vi "JLINKARM Select IP.vi"(10 "Port":i32, 11 "sHost":string) -> (3 "function return":i8)   [LabVIEW 2011, in "JLinkARM.lvlib"]
doc: "JLINKARMDLL_API char JLINKARM_SelectIP (const char* sHost, int Port);"
uses:
  Lib/JLinkARM.lvlib
  JLinkARM.dll
panel:
  out "error out":errorcluster
  in  "error in (no error)":errorcluster
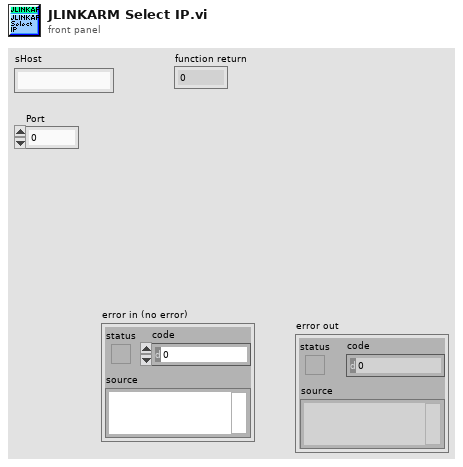
[diagram p1: front panel]
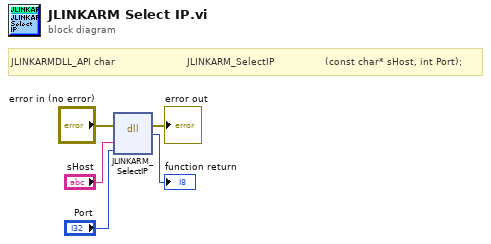
[diagram p0: block diagram]
diagram:
  # "JLINKARMDLL_API char                        JLINKARM_SelectIP                 (const char* sHost, int Port);"
  n1 = dll-call lib="C:/Documents and Settings/Anybody/Desktop/JLink_SDK_V684a/JLinkARM.*" fn="JLINKARM_SelectIP"(error in="error in (no error)", "sHost"="sHost", "Port"="Port") -> (error out=→"error out":errorcluster, →"function return":i8)  [unwired: 4 in, 1 out]
